vi "Spy Flush Errors.vi"(8 "error in (no error)":errorcluster, 11 "Mock Error Handler In":refnum<class "Mock Error Handler.lvclass">) -> (0 "error out":errorcluster, 1 "Errors":errorcluster[](array[cluster]), 2 "Locations":string[](array[string]), 3 "Mock Error Handler Out":refnum<class "Mock Error Handler.lvclass">)   [LabVIEW 2020, in "Mock Error Handler.lvclass"]
doc: "Spys on errors sent to the error handler. This Method requires a lock on the execution thread to prevent race conditions when testing other processes using the error handler."
uses:
  Mock Error Handler.lvclass
  Mock Error Handler.lvclass/Mock Error Handler.ctl
  Private/Error Message Data.ctl
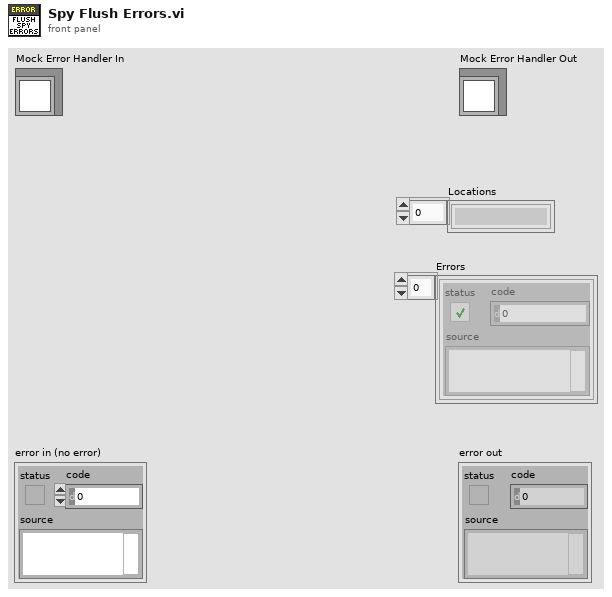
[diagram p1: front panel]
types:
  T1 = typedef "Mock Error Handler.lvclass/Error Message Data.ctl" = cluster{"Error Type":string, "Location":string, "Error":errorcluster}
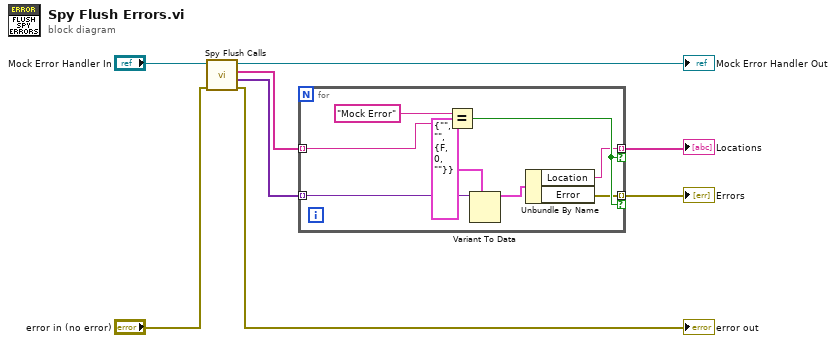
[diagram p0: block diagram]
diagram:
  n1 = call "Spy Flush Calls.vi"("error in (no error)"="error in (no error)", "Mock Process In"="Mock Error Handler In") -> ("error out"=→"error out":errorcluster, "Message Data"=w5:variant[], "Message"=w6:string[], "Mock Process Out"=→"Mock Error Handler Out":refnum<class "Mock Error Handler.lvclass">)  [unwired: 6 in]
  n2 = for {
    tunnel: [w12] -> w8 mode=indexing if=w15
    tunnel: [w9] -> w7 mode=indexing if=w15
    tunnel: w6 -> [w11] mode=indexing
    tunnel: w5 -> [w10] mode=indexing
    n3 = Equal?(x="Mock Error", y=w11) -> (x = y?=w15:bool)
    n4 = Variant To Data(type=T1 {"Error Type"="", "Location"="", "Error"={"status"=FALSE, "code"=0, "source"=""}} ("Error Message Data"), Variant=w10) -> (data=w14:T1)  [unwired: 1 in, 1 out]
    n5 = Unbundle By Name(w14) -> ("Location"=w9:string, "Error"=w12:errorcluster)
  }
  "Locations" <- w7
  "Errors" <- w8
